vi "Create doublePush move.vi"(6 "enPassant target":T1={"File"=enum."d", "Rank"=enum."4"}, 9 "Destination":T1={"File"=enum."d", "Rank"=enum."4"}, 10 "Source":T1={"File"=enum."d", "Rank"=enum."4"}) -> (3 "DoublePush move":refnum<class "DoublePush.lvclass">)   [LabVIEW 2016, in "Chesslib.lvlib" / "DoublePush.lvclass"]
uses:
  DoublePush.lvclass
  C:/Users/GRTaggJ/Documents/Projects/chesslib/Moves/Move/Move.lvclass
  typedef/Square.ctl
  typedef/File.ctl
  typedef/Rank.ctl
  DoublePush.lvclass/DoublePush.ctl
  Move/Move.lvclass
  Chesslib.lvlib
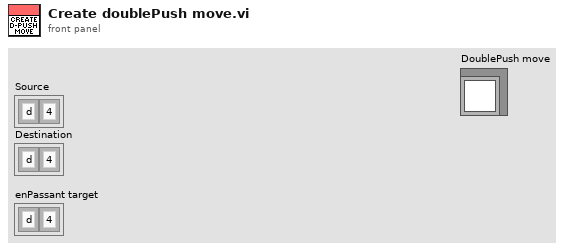
[diagram p1: front panel]
types:
  T1 = typedef "Chesslib.lvlib/Square.ctl" = cluster{"File":T2, "Rank":T3}
  T2 = typedef "Chesslib.lvlib/File.ctl" = enum8{"a", "b", "c", "d", "e", "f", "g", "h"}
  T3 = typedef "Chesslib.lvlib/Rank.ctl" = enum8{"1", "2", "3", "4", "5", "6", "7", "8"}
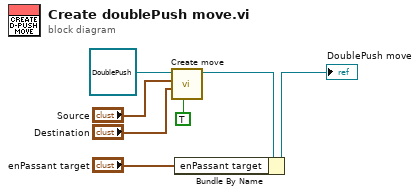
[diagram p0: block diagram]
diagram:
  n1 = call "Create move.vi"("Pawn move (F)"=TRUE, "Destination"="Destination", "Source"="Source", "Move in"=refnum<class "DoublePush.lvclass"> refnum ("DoublePush in")) -> ("Move out"=w6:refnum<class "DoublePush.lvclass">)  [unwired: 7 in]
  n2 = Bundle By Name(cluster=w6, "enPassant target"="enPassant target") -> (→"DoublePush move":refnum<class "DoublePush.lvclass">)
